vi "ACIR_DCIR_BT3562_temporaire.vi"(6 "numeroconti":u64, 7 "juste R?":bool, 8 "errin":errorcluster, 9 "chemin de base":path, 10 "section":string="Hioki BT3562", 11 "VISAin":refnum<visa-resource-name>) -> (0 "errout":errorcluster, 1 "OK?":bool, 2 "V":dbl format="%#.3f V", 3 "R":dbl format="%#_6f mOhm", 4 "LogHtml":string[](array[string]), 5 "DataStr":cluster{"Rstr":string, "Vstr":string})   [LabVIEW 2020]
uses:
  <instrlib>/HIOKI BT356X Series/Public/_Initialize/Initialize_serial.vi
  <instrlib>/HIOKI BT356X Series/Public/Action-Status/_Trigger/Init cont.vi
  <instrlib>/HIOKI BT356X Series/Public/Configure/_Trigger/Trigger.vi
  <instrlib>/HIOKI BT356X Series/Public/Configure/_Range/Voltage range.vi
  <instrlib>/HIOKI BT356X Series/Public/Configure/_Range/Resistance range.vi
  <instrlib>/HIOKI BT356X Series/HIOKI BT356X Series.lvlib
panel:
  out "Output Str":string[](array[string])
  out "LogSTD":string
  in  "bin":bool
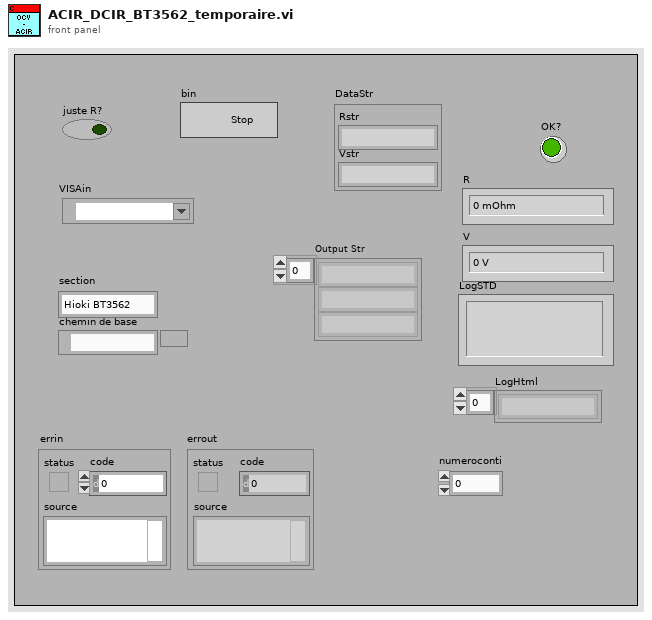
[diagram p1: front panel]
types:
  T1 = cluster{"Timeout":dbl, "Baud":u32, "Vmin":dbl, "Vmax":dbl, "RminMili":dbl, "Rmaxmili":dbl, "Vrange":dbl}
  T2 = enum32{"BT3561A", "BT3562A", "BT3563A", "BT3562", "BT3563", "BT3564", "3561"}
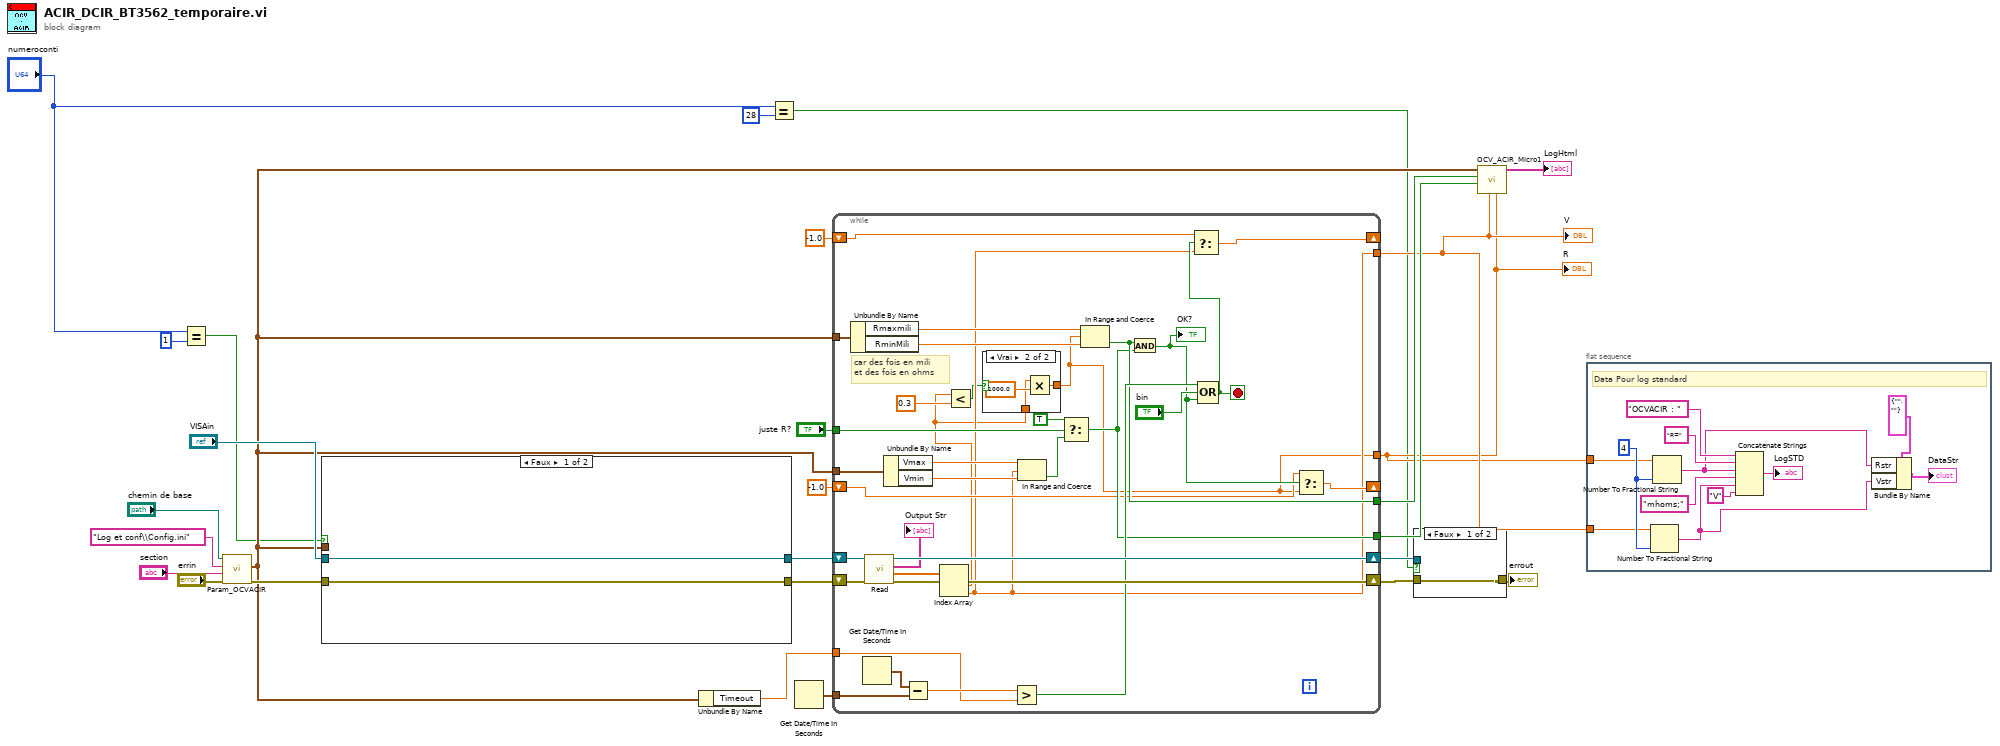
[diagram p0: block diagram]
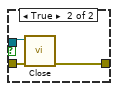
[diagram p2: hidden frame]
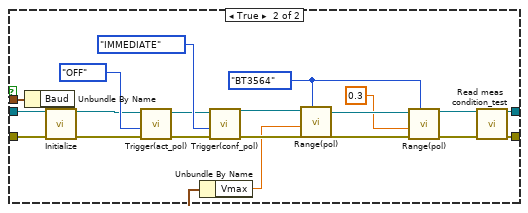
[diagram p3: hidden frame]
diagram:
  n1 = Equal?(x="numeroconti", y=u64 1) -> (x = y?=w5:bool)
  n2 = call "Param_OCVACIR.vi"("errin"="errin", "section"="section", "Chaîne"="Log et conf\\Config.ini", "pathin"="chemin de base") -> ("Errout"=w19:errorcluster, "DATA"=w10:T1)  [unwired: 6 in]
  n3 = case shown="Faux" w5 {
    tunnel: [w28 w44] -> w24
    tunnel: [w29 w43] -> w23
    tunnel: w19 -> [w28 w42]
    tunnel: "VISAin" -> [w29 w40]
    tunnel: w10 -> [_ w31]
    frame False {
    }
    frame True {
      w35 = T2."BT3564" ("Model")
      n4 = Unbundle By Name(w31) -> ("Baud"=w41:u32)
      n5 = call-poly <instrlib>:"Initialize.vi"("VISA resource name"=w40, "Baud Rate"=w41, "error in (no error)"=w42) -> ("VISA resource name out"=w46:refnum<visa-resource-name>, "error out"=w45:errorcluster)  [unwired: 11 in]
      n6 = call-poly <instrlib>:"Trigger(act_pol).vi"("error in (no error)"=w45, "Do not idle set"=enum16{"ON", "OFF"}."OFF", "VISA session"=w46) -> ("error out"=w49:errorcluster, "dup VISA session"=w48:refnum<visa-resource-name>)  [unwired: 6 in, 1 out]
      n7 = Unbundle By Name(w31) -> ("Vmax"=w30:dbl)
      n8 = call-poly <instrlib>:"Trigger(conf_pol).vi"("error in (no error)"=w49, "Trigger set"=enum16{"IMMEDIATE", "EXTERNAL"}."IMMEDIATE", "VISA session"=w48) -> ("error out"=w38:errorcluster, "dup VISA session"=w39:refnum<visa-resource-name>)  [unwired: 6 in, 1 out]
      n9 = call-poly <instrlib>:"Range(pol).vi"("Model"=w35, "error in (no error)"=w38, "Voltage Range set"=w30, "VISA session"=w39) -> ("error out"=w36:errorcluster, "dup VISA session"=w37:refnum<visa-resource-name>)  [unwired: 5 in, 1 out]
      n10 = call-poly <instrlib>:"Range(pol).vi"("Model"=w35, "error in (no error)"=w36, "Resistance range set"=0.3, "VISA session"=w37) -> ("error out"=w33:errorcluster, "dup VISA session"=w32:refnum<visa-resource-name>)  [unwired: 5 in, 1 out]
      n11 = call <instrlib>:"Read meas condition_test.vi"("VISA RefnumIn"=w32, "ErrIn"=w33) -> ("VISA Refnumo"=w43:refnum<visa-resource-name>, "Errout"=w44:errorcluster)  [unwired: 9 in, 3 out]
    }
  }
  n12 = Unbundle By Name(w10) -> ("Timeout"=w14:dbl)
  n13 = Equal?(x="numeroconti", y=u64 28) -> (x = y?=w3:bool)
  n14 = Get Date/Time In Seconds() -> (seconds since 1Jan1904=w22:timestamp)
  n15 = while {
    shift-right: [w81] -> w27
    shift-left: w23 -> [w82]
    shift-right: [w80] -> w26
    shift-left: w24 -> [w83]
    tunnel: w22 -> [w77]
    shift-right: [w73] -> _
    shift-left: -1.0 ("cas faux") -> [w57]
    shift-right: [w72] -> _
    shift-left: -1.0 ("cas faux") -> [w56]
    tunnel: [w61] -> w16
    tunnel: [w71] -> w15
    tunnel: w10 -> [w70]
    tunnel: w14 -> [w67]
    tunnel: w10 -> [w66]
    tunnel: "juste R?" -> [w63]
    tunnel: [w55] -> w7
    tunnel: [w51] -> w6
    stop <- w58 stop-if-true
    # "car des fois en mili \net des fois en ohms"
    n16 = Unbundle By Name(w66) -> ("Rmaxmili"=w65:dbl, "RminMili"=w64:dbl)
    n17 = Get Date/Time In Seconds() -> (seconds since 1Jan1904=w78:timestamp)
    n18 = call <instrlib>:"Read.vi"("error in (no error)"=w83, "VISA session"=w82) -> ("error out"=w80:errorcluster, "Output Val"=w84:dbl[], "Output Str"=→"Output Str":string[], "dup VISA session"=w81:refnum<visa-resource-name>)  [unwired: 6 in]
    n19 = Unbundle By Name(w70) -> ("Vmax"=w69:dbl, "Vmin"=w68:dbl)
    n20 = Subtract(x=w78, y=w77) -> (x-y=w76:dbl)
    n21 = Index Array(array=w84) -> (element #1=w52:dbl, element #2=w55:dbl)  [unwired: 2 in]
    n22 = Less?(x=w52, y=0.3) -> (x < y?=w53:bool)
    n23 = case shown="Vrai" w53 {
      tunnel: w52 -> [w85 w87]
      tunnel: [w85 w86] -> w51
      frame False {
      }
      frame True {
        n24 = Multiply(x=w87, y=1000.0) -> (x*y=w86:dbl)
      }
    }
    n25 = Greater?(x=w76, y=w67) -> (0:w75:bool)
    n26 = In Range and Coerce(upper limit=w69, x=w55, lower limit=w68) -> (In Range?=w62:bool)  [unwired: 1 out]
    n27 = Select(t=TRUE ("cas vrai"), s=w63, f=w62) -> (s? t:f=w61:bool)
    n28 = In Range and Coerce(upper limit=w65, x=w51, lower limit=w64) -> (In Range?=w71:bool)  [unwired: 1 out]
    n29 = And(x=w71, y=w61) -> (x .and. y?=w74:bool)
    "OK?" <- w74
    n30 = Compound Arithmetic op=OR ("Opérateur arithmétique")(w75, "bin", w74) -> (w58:bool)
    n31 = Select(t=w57, s=w58, f=w55) -> (s? t:f=w73:dbl)
    n32 = Select(t=w56, s=w74, f=w51) -> (s? t:f=w72:dbl)
  }
  "R" <- w6
  "V" <- w7
  n33 = case shown="Faux" w3 {
    tunnel: w27 -> [_ w92]
    tunnel: w26 -> [w89 w91]
    tunnel: [w89 w90] -> w25
    frame False {
    }
    frame True {
      n34 = call <instrlib>:"Close.vi"("error in (no error)"=w91, "VISA resource name"=w92) -> ("error out"=w90:errorcluster)  [unwired: 9 in]
    }
  }
  "errout" <- w25
  n35 = call "OCV_ACIR_Micro1.vi"("R"=w6, "V"=w7, "V OK"=w16, "R OK"=w15, "DATA"=w10) -> ("Tableau"=→"LogHtml":string[])  [unwired: 6 in]
  n36 = flat-sequence {
    tunnel: w6 -> [w98]
    tunnel: w7 -> [w97]
    frame #0 {
      w104 = i16 4 ("précision (6)")
      # "Data Pour log standard"
      n37 = Number To Fractional String(number=w97, precision (6)=w104) -> (F-format string=w93:string)  [unwired: 2 in]
      n38 = Number To Fractional String(number=w98, precision (6)=w104) -> (F-format string=w94:string)  [unwired: 2 in]
      n39 = Concatenate Strings("OCVACIR : " ("chaîne"), "R=" ("chaîne"), w94, "mhoms;" ("chaîne"), w93, "V" ("chaîne")) -> (→"LogSTD":string)
      n40 = Bundle By Name(cluster=cluster{"Rstr":string, "Vstr":string} {"Rstr"="", "Vstr"=""} ("DataStr"), "Rstr"=w94, "Vstr"=w93) -> (→"DataStr":cluster{"Rstr":string, "Vstr":string})
    }
  }
